vi "read_tiff_header.vi"() -> ()   [LabVIEW 2013]
uses:
  <vilib>/vision/NI_Vision_Development_Module.lvlib
  <vilib>/Analysis/NI_AALPro.lvlib
panel:
  in  "Tab Control":enum32{"Page 1", "Page2", "Page 3", "Page 4"}(tab)
  out "Image":T1(plugin-control)
  out "byte order":T2(ring)
  out "version":u16 format="%x"
  out "byteorder":u16 format="%x"
  in  "frame_index":i32(listbox)
  in  "Directory Entry_index":i32(listbox)
  in  "DE_Data":T3(tab)
  out "type1":u8[](array[numeric])
  out "type2":string
  out "type3":u16[](array[numeric])
  out "type4":u32[](array[numeric])
  out "type5":u32[](array[numeric])
  out "BitDeepth":u32
  out "ImagerWidth":u32
  out "ImageLength":u32
  out "Histogram Graph":T4(graph)
  in  "16-bit Display Mapping:All Elements":T5={"Conversion Method"=2, "Minimum Value"=-30, "Maximum Value"=225, "Number Of Shifts"=0}
  out "tag_ID":u16 format="%x"
  out "DE_data_num":u32
  out "type_ID":u16 format="%x"
  out "DE_data_offset":u32
  out "current_DE_offset":u32 format="%x"
  out "current_IFD_offset":u32 format="%x"
  out "DE_tag_IDs":u16[](array[numeric]) format="%x"
  out "RowsPerStrip":u32
  out "StripByteCounts":u32[](array[numeric])
  out "output array":i32[][](array[numeric])
  out "file header":T6 {"byteorder" format="%x"; "version" format="%x"; "Offset_first_IFD" format="%x"}
  out "DE_num":u16 format="%x"
  out "index of RowsPerStrip":i32
  out "index of bitdeepth":i32
  out "index of StripByteCounts":i32
  out "index of StripOffsets":i32
  out "index of ImageLength":i32
  out "index of ImageWidth":i32
  out "StripOffsets":u32[](array[numeric]) format="%x"
  out "IFD_offset_Array":u32[](array[numeric]) format="%x"
  in  "open":bool
  out "type2_char":string
  out "type1_U8":u8
  out "type4_U32":u32
  out "type5_RATIONAL":u32
  out "type3_U16":u16
  out "selected path":path
  out "tif_file":refnum<file>
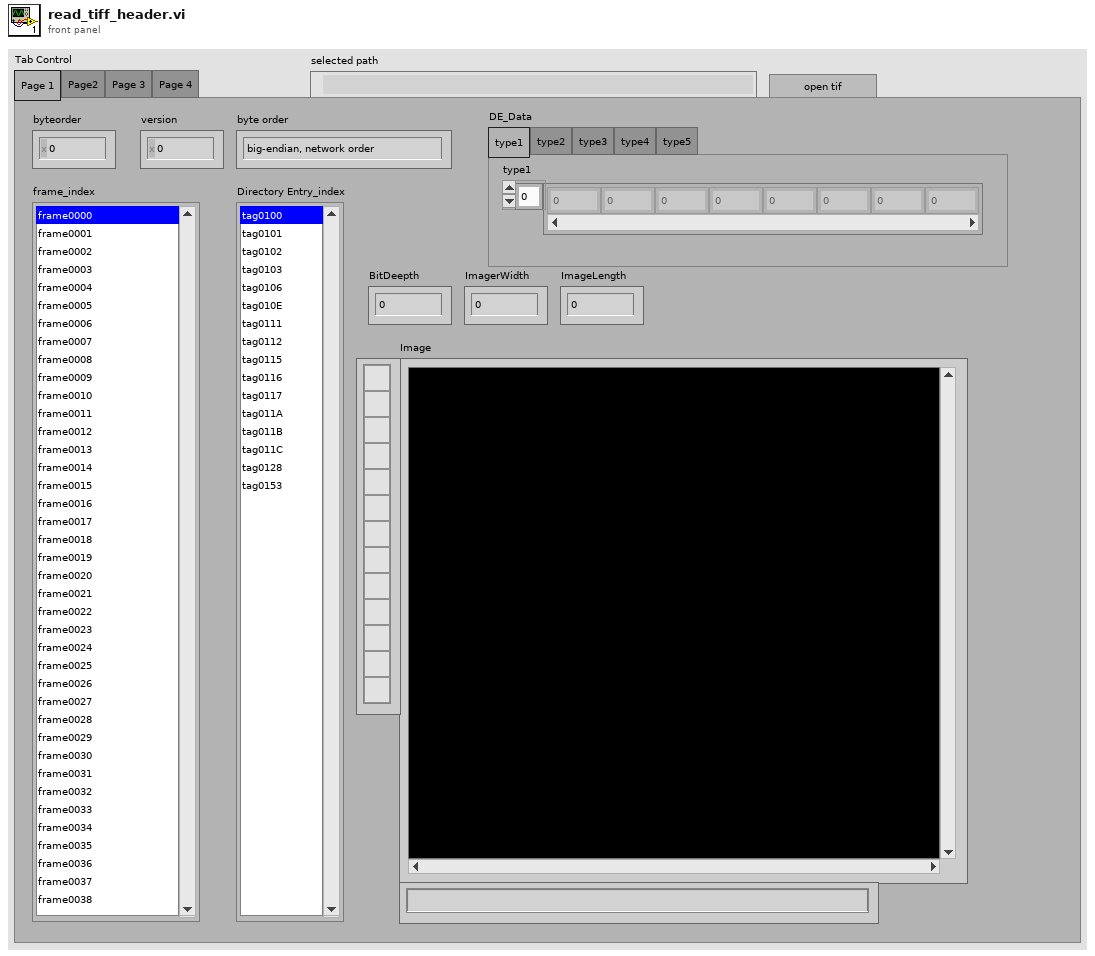
[diagram p1: front panel]
types:
  T1 = typedef "IMAQ Image.ctl" = refnum<image>
  T2 = enum16{"big-endian, network order", "native, host order", "little-endian"}
  T3 = enum32{"type1", "type2", "type3", "type4", "type5"}
  T4 = cluster{"X Values":dbl[], "Histogram: h(x)":i32[]}
  T5 = cluster{"Conversion Method":u32, "Minimum Value":i32, "Maximum Value":i32, "Number Of Shifts":i32}
  T6 = cluster{"byteorder":u16, "version":u16, "Offset_first_IFD":u32}
  T7 = cluster{"tag_ID":u16, "type_ID":u16, "DE_data_num":u32, "DE_data_offset":u32, "type1":u8[], "type2":string, "type3":u16[], "type4":u32[], "type5":u32[]}
  T8 = typedef "Image Type" = u32
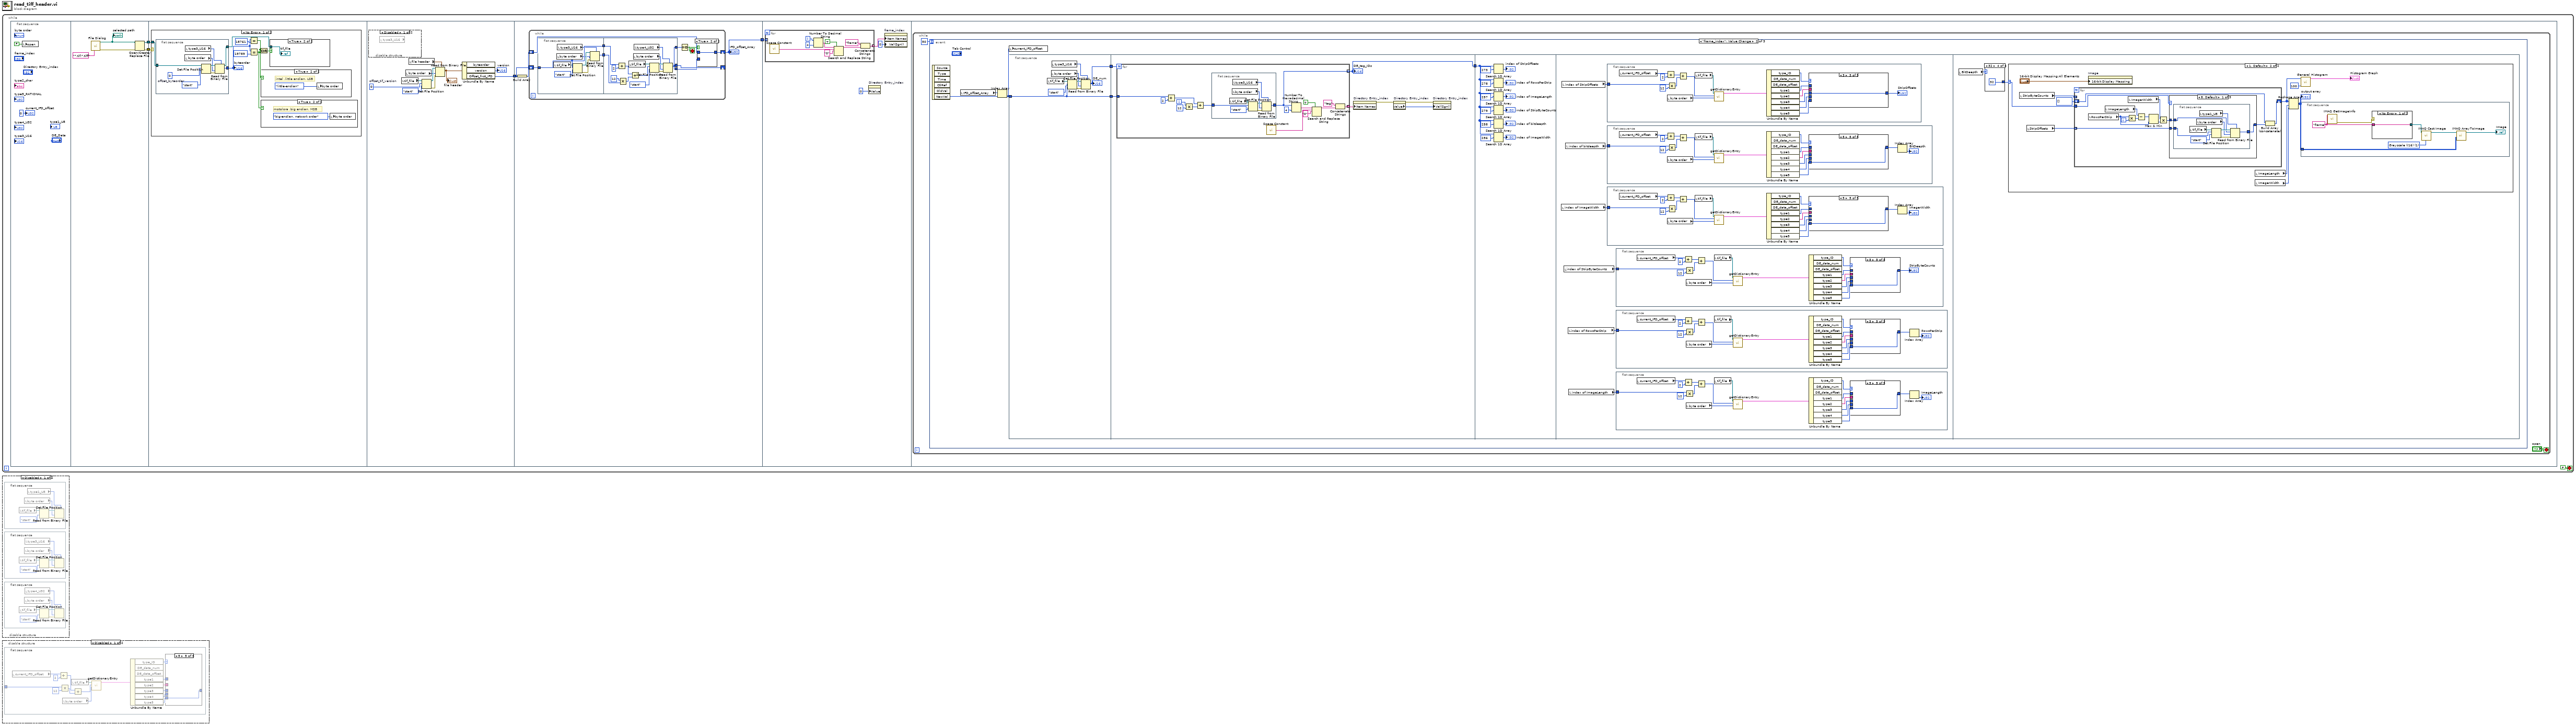
[diagram p0: block diagram]
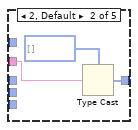
[diagram p3: hidden frame]
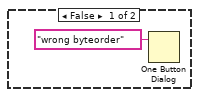
[diagram p7: hidden frame]
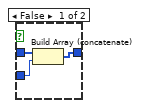
[diagram p12: hidden frame]
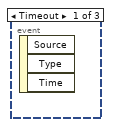
[diagram p13: hidden frame]
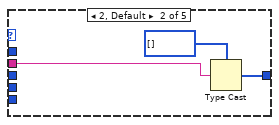
[diagram p15: hidden frame]
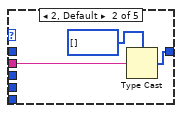
[diagram p19: hidden frame]
diagram:
  n1 = while {
    stop <- FALSE stop-if-true
    n2 = flat-sequence {
      tunnel: [w9] -> w5
      tunnel: [w8] -> w2
      tunnel: w5 -> [w14]
      tunnel: w2 -> [w13]
      tunnel: [w36] -> w1
      tunnel: [w47] -> w4
      tunnel: w1 -> [w46]
      tunnel: w4 -> [w87]
      frame #0 {
        n3 = local write "open"(FALSE ("Stop Button")) -> ()
        "current_IFD_offset" <- u32 0 ("current_IFD_offset")
      }
      frame #1 {
        n4 = call "File Dialog"("pattern (all files)"="*.tif;*.tiff") -> ("selected path"=w10:path, "error out"=w12:errorcluster)  [unwired: 11 in, 2 out]
        "selected path" <- w10
        n5 = Open/Create/Replace File(file path (use dialog)=w10, error in=w12) -> (refnum out=w8:refnum<file>, error out=w9:errorcluster)  [unwired: 4 in, 1 out]
      }
      frame #2 {
        n6 = case shown="No Error" w14 {
          tunnel: w13 -> [w17 _]
          frame No Error {
            n7 = flat-sequence {
              tunnel: [w26] -> w15
              tunnel: w17 -> [w25]
              tunnel: [w24] -> w16
              frame #0 {
                w27 = i64 0  # offset_byteorder
                n8 = local read "byte order"() -> (w28:T2)
                n9 = local read "type3_U16"() -> (w23:u16)
                n10 = Set File Position(offset (in bytes) (0)=w27, refnum=w25, from (0:start)=enum16{"start", "end", "current"}."start") -> (refnum out=w29:refnum<file>, error out=w30:errorcluster)  [unwired: 1 in]
                n11 = Read from Binary File(5:w23, 8:w30, 9:w28, 11:w29) -> (2:w26:u16, 3:w24:refnum<file>)  [unwired: 2 in, 2 out]
              }
            }
            n12 = Equal?(x=w15, y=u16 18761) -> (x = y?=w20:bool)
            n13 = Equal?(x=w15, y=u16 19789) -> (x = y?=w19:bool)
            n14 = Or(x=w20, y=w19) -> (x .or. y?=w18:bool)
            n15 = case shown="True" w20 {
              frame False {
              }
              frame True {
                # "intel ,little endian, LSB"
                n16 = local write "byte order"(T2."little-endian" ("byte order")) -> ()
              }
            }
            n17 = case shown="True" w19 {
              frame False {
              }
              frame True {
                # "motolora ,big endian, MSB"
                n18 = local write "byte order"(T2."big-endian, network order" ("byte order")) -> ()
              }
            }
            n19 = case shown="True" w18 {
              tunnel: w16 -> [_ w33]
              frame False {
                n20 = One Button Dialog(message="wrong byteorder") -> ()  [unwired: 1 in, 1 out]
              }
              frame True {
                "tif_file" <- w33
              }
            }
            "byteorder" <- w15
          }
          frame Error {
          }
        }
      }
      frame #3 {
        w40 = i64 0  # offset_tif_version
        n21 = disable-structure shown="Disabled" {
          frame Disabled {
            n22 = local read "type3_U16"() -> ()  [unwired: 1 out]
          }
          frame Enabled {
          }
        }
        n23 = local read "tif_file"() -> (w45:refnum<file>)
        n24 = local read "byte order"() -> (w41:T2)
        n25 = local read "file header"() -> (w39:T6)
        n26 = Set File Position(offset (in bytes) (0)=w40, refnum=w45, from (0:start)=enum16{"start", "end", "current"}."start") -> (refnum out=w42:refnum<file>, error out=w43:errorcluster)  [unwired: 1 in]
        n27 = Read from Binary File(5:w39, 8:w43, 9:w41, 11:w42) -> (2:w38:T6)  [unwired: 2 in, 3 out]
        "file header" <- w38
        n28 = Unbundle By Name(w38) -> ("version"=→"version":u16, "Offset_first_IFD"=w36:u32)  [unwired: 1 out]
      }
      frame #4 {
        n29 = Build Array(w46) -> (w48:u32[])
        n30 = while {
          shift-right: [w55] -> _
          shift-left: w46 -> [w57]
          shift-right: [w50] -> w47
          shift-left: w48 -> [w51]
          stop <- w49 stop-if-true
          n31 = flat-sequence {
            tunnel: w57 -> [w68]
            tunnel: [w69] -> w54
            tunnel: [w68] -> w53
            tunnel: [w70] -> w56
            tunnel: [w70] -> w55
            tunnel: w54 -> [w72]
            tunnel: w53 -> [w71]
            tunnel: [w70] -> w52
            frame #0 {
              n32 = local read "tif_file"() -> (w67:refnum<file>)
              n33 = local read "byte order"() -> (w63:T2)
              n34 = local read "type3_U16"() -> (w62:u16)
              n35 = Set File Position(offset (in bytes) (0)=w68, refnum=w67, from (0:start)=enum16{"start", "end", "current"}."start") -> (refnum out=w64:refnum<file>, error out=w65:errorcluster)  [unwired: 1 in]
              n36 = Read from Binary File(5:w62, 8:w65, 9:w63, 11:w64) -> (2:w69:u16)  [unwired: 2 in, 3 out]
            }
            frame #1 {
              n37 = Add(x=w71, y=u32 2) -> (x+y=w75:u32)
              n38 = Multiply(x=u16 12 ("y"), y=w72) -> (x*y=w74:u16)
              n39 = local read "tif_file"() -> (w83:refnum<file>)
              n40 = Add(x=w75, y=w74) -> (x+y=w73:u32)
              n41 = local read "byte order"() -> (w79:T2)
              n42 = local read "type4_U32"() -> (w78:u32)
              n43 = Set File Position(offset (in bytes) (0)=w73, refnum=w83, from (0:start)=enum16{"start", "end", "current"}."start") -> (refnum out=w80:refnum<file>, error out=w81:errorcluster)  [unwired: 1 in]
              n44 = Read from Binary File(5:w78, 8:w81, 9:w79, 11:w80) -> (2:w70:u32)  [unwired: 2 in, 3 out]
            }
          }
          n45 = Equal To 0?(x=w56) -> (x = 0?=w49:bool)
          n46 = case shown="True" w49 {
            tunnel: w52 -> [w60 _]
            tunnel: w51 -> [w59 w61]
            tunnel: [w58 w61] -> w50
            frame False {
              n47 = Build Array (concatenate)(w59, w60) -> (w58:u32[])
            }
            frame True {
            }
          }
        }
        "IFD_offset_Array" <- w47
      }
      frame #5 {
        n48 = for {
          tunnel: w87 -> [_] mode=indexing
          tunnel: [w90] -> w86 mode=indexing
          i -> [w96]
          n49 = call <vilib>:"Space Constant.vi"() -> ("String"=w92:string)
          n50 = Number To Decimal String(number=w96, width (-)=i16 4) -> (decimal integer string=w93:string)
          n51 = Search and Replace String(replace all?=TRUE ("replace all? (F)"), input string=w93, search string=w92, replace string="0" ("replace string (\"\")")) -> (result string=w88:string)  [unwired: 4 in, 3 out]
          n52 = Concatenate Strings("frame" ("string"), w88) -> (w90:string)
        }
        n53 = property on="Directory Entry_index" class="LstBox (strict)"("Value"=0 ("Value (Signaling)")) -> ()  [unwired: 2 in, 2 out]
        n54 = property on="frame_index" class="LstBox (strict)"("Item Names"=w86, "Val(Sgnl)"=0 ("Value (Signaling)")) -> ()  [unwired: 2 in, 2 out]
      }
      frame #6 {
        n55 = while {
          stop <- "open" stop-if-true
          n56 = event shown="[1] \"frame_index\": Value Change" {
            selector: _ -> [_ _ _]
            dyn-events: _ -> [_ _ _]
            timeout: 50 -> [_ _ _]
            event Timeout {
              n57 = event-data() -> ()  [unwired: 1 in, 3 out]
            }
            event "frame_index": Value Change {
              n58 = event-data() -> ("NewVal"=w103:i32)  [unwired: 1 in, 5 out]
              n59 = local read "IFD_offset_Array"() -> (w104:u32[])
              n60 = Index Array(array=w104, index=w103) -> (element=w102:u32)
              n61 = local write "current_IFD_offset"(w102) -> ()
              n62 = flat-sequence {
                tunnel: w102 -> [w105]
                tunnel: [w106] -> w101
                tunnel: [w105] -> w100
                tunnel: w101 -> [w119]
                tunnel: w100 -> [w114]
                tunnel: [w113] -> w99
                tunnel: w99 -> [w144]
                frame #0 {
                  n63 = local read "tif_file"() -> (w112:refnum<file>)
                  n64 = local read "byte order"() -> (w108:T2)
                  n65 = local read "type3_U16"() -> (w107:u16)
                  n66 = Set File Position(offset (in bytes) (0)=w105, refnum=w112, from (0:start)=enum16{"start", "end", "current"}."start") -> (refnum out=w109:refnum<file>, error out=w110:errorcluster)  [unwired: 1 in]
                  n67 = Read from Binary File(5:w107, 8:w110, 9:w108, 11:w109) -> (2:w106:u16)  [unwired: 2 in, 3 out]
                  "DE_num" <- w106
                }
                frame #1 {
                  n68 = for {
                    N: w119 -> [_]
                    tunnel: [w128] -> w118 mode=indexing
                    tunnel: w114 -> [w127]
                    tunnel: [w120] -> w113 mode=indexing
                    i -> [w125]
                    n69 = Add(x=w127, y=u32 2) -> (x+y=w123:u32)
                    n70 = Multiply(x=w125, y=12) -> (x*y=w122:i32)
                    n71 = Add(x=w123, y=w122) -> (x+y=w121:u32)
                    n72 = flat-sequence {
                      tunnel: w121 -> [w137]
                      tunnel: [w136] -> w120
                      frame #0 {
                        n73 = local read "tif_file"() -> (w143:refnum<file>)
                        n74 = local read "byte order"() -> (w139:T2)
                        n75 = local read "type3_U16"() -> (w138:u16)
                        n76 = Set File Position(offset (in bytes) (0)=w137, refnum=w143, from (0:start)=enum16{"start", "end", "current"}."start") -> (refnum out=w140:refnum<file>, error out=w141:errorcluster)  [unwired: 1 in]
                        n77 = Read from Binary File(5:w138, 8:w141, 9:w139, 11:w140) -> (2:w136:u16)  [unwired: 2 in, 3 out]
                      }
                    }
                    n78 = call <vilib>:"Space Constant.vi"() -> ("String"=w132:string)
                    n79 = Number To Hexadecimal String(1:i16 4 ("width (-)"), 2:w120) -> (0:w133:string)
                    n80 = Search and Replace String(replace all?=TRUE ("replace all? (F)"), input string=w133, search string=w132, replace string="0" ("replace string (\"\")")) -> (result string=w129:string)  [unwired: 4 in, 3 out]
                    n81 = Concatenate Strings("tag" ("string"), w129) -> (w128:string)
                  }
                  "DE_tag_IDs" <- w113
                  n82 = property on="Directory Entry_index" class="LstBox (strict)"("Item Names"=w118) -> (error out=w116:errorcluster)  [unwired: 2 in, 1 out]
                  n83 = property on="Directory Entry_index" class="LstBox (strict)"(error in=w116) -> (error out=w115:errorcluster, "Value"=w117:i32)  [unwired: 1 in, 1 out]
                  n84 = property on="Directory Entry_index" class="LstBox (strict)"(error in=w115, "Val(Sgnl)"=w117) -> ()  [unwired: 1 in, 2 out]
                }
                frame #2 {
                  n85 = Search 1D Array(1D array=w144, element=u16 273) -> (index of element=→"index of StripOffsets":i32)  [unwired: 1 in]
                  n86 = Search 1D Array(1D array=w144, element=u16 278) -> (index of element=→"index of RowsPerStrip":i32)  [unwired: 1 in]
                  n87 = Search 1D Array(1D array=w144, element=u16 257) -> (index of element=→"index of ImageLength":i32)  [unwired: 1 in]
                  n88 = Search 1D Array(1D array=w144, element=u16 279) -> (index of element=→"index of StripByteCounts":i32)  [unwired: 1 in]
                  n89 = Search 1D Array(1D array=w144, element=u16 258) -> (index of element=→"index of bitdeepth":i32)  [unwired: 1 in]
                  n90 = Search 1D Array(1D array=w144, element=u16 256) -> (index of element=→"index of ImageWidth":i32)  [unwired: 1 in]
                }
                frame #3 {
                  n91 = local read "index of ImageWidth"() -> (w159:i32)
                  n92 = local read "index of StripOffsets"() -> (w157:i32)
                  n93 = local read "index of StripByteCounts"() -> (w160:i32)
                  n94 = local read "index of bitdeepth"() -> (w162:i32)
                  n95 = local read "index of RowsPerStrip"() -> (w161:i32)
                  n96 = local read "index of ImageLength"() -> (w158:i32)
                  n97 = flat-sequence {
                    tunnel: w157 -> [w177]
                    frame #0 {
                      n98 = local read "current_IFD_offset"() -> (w179:u32)
                      n99 = Add(x=w179, y=2) -> (x+y=w175:u32)
                      n100 = local read "byte order"() -> (w171:T2)
                      n101 = Multiply(x=w177, y=12) -> (x*y=w174:i32)
                      n102 = Add(x=w175, y=w174) -> (x+y=w173:u32)
                      n103 = local read "tif_file"() -> (w172:refnum<file>)
                      n104 = call "getDictionaryEntry.vi"("byte order"=w171, "DE_offset"=w173, "tif_file"=w172) -> ("output cluster"=w170:T7)  [unwired: 7 in, 1 out]
                      n105 = Unbundle By Name(w170) -> ("type_ID"=w169:u16, "type1"=w168:u8[], "type2"=w164:string, "type3"=w167:u16[], "type4"=w166:u32[], "type5"=w165:u32[])  [unwired: 2 out]
                      n106 = case shown="3" w169 {
                        tunnel: [w180 w181 w184 w185 w186] -> w163
                        tunnel: w168 -> [w180 _ _ _ _]
                        tunnel: w167 -> [_ _ w184 _ _]
                        tunnel: w166 -> [_ _ _ w185 _]
                        tunnel: w165 -> [_ _ _ _ w186]
                        tunnel: w164 -> [_ w183 _ _ _]
                        frame 1 {
                        }
                        frame 2, Default {
                          n107 = Type Cast(type=u8[] [] ("type1"), x=w183) -> (*(type *) &x=w181:u8[])
                        }
                        frame 3 {
                        }
                        frame 4 {
                        }
                        frame 5 {
                        }
                      }
                      "StripOffsets" <- w163
                    }
                  }
                  n108 = flat-sequence {
                    tunnel: w162 -> [w301]
                    frame #0 {
                      n109 = local read "current_IFD_offset"() -> (w303:u32)
                      n110 = Add(x=w303, y=2) -> (x+y=w299:u32)
                      n111 = local read "byte order"() -> (w295:T2)
                      n112 = Multiply(x=w301, y=12) -> (x*y=w298:i32)
                      n113 = Add(x=w299, y=w298) -> (x+y=w297:u32)
                      n114 = local read "tif_file"() -> (w296:refnum<file>)
                      n115 = call "getDictionaryEntry.vi"("byte order"=w295, "DE_offset"=w297, "tif_file"=w296) -> ("output cluster"=w294:T7)  [unwired: 7 in, 1 out]
                      n116 = Unbundle By Name(w294) -> ("type_ID"=w293:u16, "type1"=w292:u8[], "type2"=w288:string, "type3"=w291:u16[], "type4"=w290:u32[], "type5"=w289:u32[])  [unwired: 2 out]
                      n117 = case shown="5" w293 {
                        tunnel: [w304 w305 w308 w309 w310] -> w287
                        tunnel: w292 -> [w304 _ _ _ _]
                        tunnel: w291 -> [_ _ w308 _ _]
                        tunnel: w290 -> [_ _ _ w309 _]
                        tunnel: w289 -> [_ _ _ _ w310]
                        tunnel: w288 -> [_ w307 _ _ _]
                        frame 1 {
                        }
                        frame 2, Default {
                          n118 = Type Cast(type=u8[] [] ("type1"), x=w307) -> (*(type *) &x=w305:u8[])
                        }
                        frame 3 {
                        }
                        frame 4 {
                        }
                        frame 5 {
                        }
                      }
                      n119 = Index Array(array=w287) -> (element=→"BitDeepth":u32)  [unwired: 1 in]
                    }
                  }
                  n120 = flat-sequence {
                    tunnel: w159 -> [w227]
                    frame #0 {
                      n121 = local read "current_IFD_offset"() -> (w229:u32)
                      n122 = Add(x=w229, y=2) -> (x+y=w225:u32)
                      n123 = local read "byte order"() -> (w221:T2)
                      n124 = Multiply(x=w227, y=12) -> (x*y=w224:i32)
                      n125 = Add(x=w225, y=w224) -> (x+y=w223:u32)
                      n126 = local read "tif_file"() -> (w222:refnum<file>)
                      n127 = call "getDictionaryEntry.vi"("byte order"=w221, "DE_offset"=w223, "tif_file"=w222) -> ("output cluster"=w220:T7)  [unwired: 7 in, 1 out]
                      n128 = Unbundle By Name(w220) -> ("type_ID"=w219:u16, "type1"=w218:u8[], "type2"=w214:string, "type3"=w217:u16[], "type4"=w216:u32[], "type5"=w215:u32[])  [unwired: 2 out]
                      n129 = case shown="5" w219 {
                        tunnel: [w230 w231 w234 w235 w236] -> w213
                        tunnel: w218 -> [w230 _ _ _ _]
                        tunnel: w217 -> [_ _ w234 _ _]
                        tunnel: w216 -> [_ _ _ w235 _]
                        tunnel: w215 -> [_ _ _ _ w236]
                        tunnel: w214 -> [_ w233 _ _ _]
                        frame 1 {
                        }
                        frame 2, Default {
                          n130 = Type Cast(type=u8[] [] ("type1"), x=w233) -> (*(type *) &x=w231:u8[])
                        }
                        frame 3 {
                        }
                        frame 4 {
                        }
                        frame 5 {
                        }
                      }
                      n131 = Index Array(array=w213) -> (element=→"ImagerWidth":u32)  [unwired: 1 in]
                    }
                  }
                  n132 = flat-sequence {
                    tunnel: w160 -> [w251]
                    frame #0 {
                      n133 = local read "current_IFD_offset"() -> (w253:u32)
                      n134 = Add(x=w253, y=2) -> (x+y=w249:u32)
                      n135 = Multiply(x=w251, y=12) -> (x*y=w248:i32)
                      n136 = local read "byte order"() -> (w245:T2)
                      n137 = Add(x=w249, y=w248) -> (x+y=w247:u32)
                      n138 = local read "tif_file"() -> (w246:refnum<file>)
                      n139 = call "getDictionaryEntry.vi"("byte order"=w245, "DE_offset"=w247, "tif_file"=w246) -> ("output cluster"=w244:T7)  [unwired: 7 in, 1 out]
                      n140 = Unbundle By Name(w244) -> ("type_ID"=w243:u16, "type1"=w242:u8[], "type2"=w238:string, "type3"=w241:u16[], "type4"=w240:u32[], "type5"=w239:u32[])  [unwired: 2 out]
                      n141 = case shown="5" w243 {
                        tunnel: [w254 w255 w258 w259 w260] -> w237
                        tunnel: w242 -> [w254 _ _ _ _]
                        tunnel: w241 -> [_ _ w258 _ _]
                        tunnel: w240 -> [_ _ _ w259 _]
                        tunnel: w239 -> [_ _ _ _ w260]
                        tunnel: w238 -> [_ w257 _ _ _]
                        frame 1 {
                        }
                        frame 2, Default {
                          n142 = Type Cast(type=u8[] [] ("type1"), x=w257) -> (*(type *) &x=w255:u8[])
                        }
                        frame 3 {
                        }
                        frame 4 {
                        }
                        frame 5 {
                        }
                      }
                      "StripByteCounts" <- w237
                    }
                  }
                  n143 = flat-sequence {
                    tunnel: w161 -> [w276]
                    frame #0 {
                      n144 = local read "current_IFD_offset"() -> (w278:u32)
                      n145 = Add(x=w278, y=2) -> (x+y=w274:u32)
                      n146 = Multiply(x=w276, y=12) -> (x*y=w273:i32)
                      n147 = local read "byte order"() -> (w270:T2)
                      n148 = Add(x=w274, y=w273) -> (x+y=w272:u32)
                      n149 = local read "tif_file"() -> (w271:refnum<file>)
                      n150 = call "getDictionaryEntry.vi"("byte order"=w270, "DE_offset"=w272, "tif_file"=w271) -> ("output cluster"=w269:T7)  [unwired: 7 in, 1 out]
                      n151 = Unbundle By Name(w269) -> ("type_ID"=w268:u16, "type1"=w267:u8[], "type2"=w263:string, "type3"=w266:u16[], "type4"=w265:u32[], "type5"=w264:u32[])  [unwired: 2 out]
                      n152 = case shown="5" w268 {
                        tunnel: [w279 w280 w283 w284 w285] -> w262
                        tunnel: w267 -> [w279 _ _ _ _]
                        tunnel: w266 -> [_ _ w283 _ _]
                        tunnel: w265 -> [_ _ _ w284 _]
                        tunnel: w264 -> [_ _ _ _ w285]
                        tunnel: w263 -> [_ w282 _ _ _]
                        frame 1 {
                        }
                        frame 2, Default {
                          n153 = Type Cast(type=u8[] [] ("type1"), x=w282) -> (*(type *) &x=w280:u8[])
                        }
                        frame 3 {
                        }
                        frame 4 {
                        }
                        frame 5 {
                        }
                      }
                      n154 = Index Array(array=w262) -> (element=→"RowsPerStrip":u32)  [unwired: 1 in]
                    }
                  }
                  n155 = flat-sequence {
                    tunnel: w158 -> [w202]
                    frame #0 {
                      n156 = local read "current_IFD_offset"() -> (w204:u32)
                      n157 = Add(x=w204, y=2) -> (x+y=w200:u32)
                      n158 = Multiply(x=w202, y=12) -> (x*y=w199:i32)
                      n159 = local read "byte order"() -> (w196:T2)
                      n160 = Add(x=w200, y=w199) -> (x+y=w198:u32)
                      n161 = local read "tif_file"() -> (w197:refnum<file>)
                      n162 = call "getDictionaryEntry.vi"("byte order"=w196, "DE_offset"=w198, "tif_file"=w197) -> ("output cluster"=w195:T7)  [unwired: 7 in, 1 out]
                      n163 = Unbundle By Name(w195) -> ("type_ID"=w194:u16, "type1"=w193:u8[], "type2"=w189:string, "type3"=w192:u16[], "type4"=w191:u32[], "type5"=w190:u32[])  [unwired: 2 out]
                      n164 = case shown="5" w194 {
                        tunnel: [w205 w206 w209 w210 w211] -> w188
                        tunnel: w193 -> [w205 _ _ _ _]
                        tunnel: w192 -> [_ _ w209 _ _]
                        tunnel: w191 -> [_ _ _ w210 _]
                        tunnel: w190 -> [_ _ _ _ w211]
                        tunnel: w189 -> [_ w208 _ _ _]
                        frame 1 {
                        }
                        frame 2, Default {
                          n165 = Type Cast(type=u8[] [] ("type1"), x=w208) -> (*(type *) &x=w206:u8[])
                        }
                        frame 3 {
                        }
                        frame 4 {
                        }
                        frame 5 {
                        }
                      }
                      n166 = Index Array(array=w188) -> (element=→"ImageLength":u32)  [unwired: 1 in]
                    }
                  }
                }
                frame #4 {
                  n167 = local read "BitDeepth"() -> (w312:u32)
                  n168 = case shown="32" w312 {
                    tunnel: [0 8 16 32] -> w311
                    frame 0, Default {
                    }
                    frame 8 {
                    }
                    frame 16 {
                    }
                    frame 32 {
                    }
                  }
                  n169 = case shown="1, Default" w311 {
                    selector: w311 -> [_ w321]
                    frame 0 {
                    }
                    frame 1, Default {
                      n170 = local read "StripByteCounts"() -> (w323:u32[])
                      n171 = local read "StripOffsets"() -> (w322:u32[])
                      n172 = for {
                        tunnel: w323 -> [_] mode=indexing
                        tunnel: w322 -> [w339] mode=indexing
                        tunnel: w321 -> [w335]
                        shift-right: [w336] -> w316
                        shift-left: i32[] [] -> [w337]
                        i -> [w345]
                        n173 = local read "RowsPerStrip"() -> (w342:u32)
                        n174 = local read "ImageLength"() -> (w343:u32)
                        n175 = Multiply(x=w342, y=w345) -> (x*y=w344:u32)
                        n176 = local read "ImagerWidth"() -> (w346:u32)
                        n177 = Subtract(x=w343, y=w344) -> (x-y=w340:u32)
                        n178 = Max & Min(x=w340, y=w342) -> (min(x,y)=w341:u32)  [unwired: 1 out]
                        n179 = Multiply(x=w346, y=w341) -> (x*y=w334:u32)
                        n180 = case shown="8, Default" w335 {
                          tunnel: w339 -> [w349 w361 w373]
                          tunnel: [w347 w359 w372] -> w338
                          tunnel: w334 -> [w348 w360 w371]
                          frame 8, Default {
                            n181 = flat-sequence {
                              tunnel: w349 -> [w352]
                              tunnel: w348 -> [w351]
                              tunnel: [w350] -> w347
                              frame #0 {
                                n182 = local read "tif_file"() -> (w358:refnum<file>)
                                n183 = local read "byte order"() -> (w354:T2)
                                n184 = local read "type1_U8"() -> (w353:u8)
                                n185 = Set File Position(offset (in bytes) (0)=w352, refnum=w358, from (0:start)=enum16{"start", "end", "current"}."start") -> (refnum out=w355:refnum<file>, error out=w356:errorcluster)  [unwired: 1 in]
                                n186 = Read from Binary File(5:w353, 8:w356, 9:w354, 10:w351, 11:w355) -> (2:w350:u8[])  [unwired: 1 in, 3 out]
                              }
                            }
                          }
                          frame 16 {
                            n187 = flat-sequence {
                              tunnel: w361 -> [w365]
                              tunnel: w360 -> [w364]
                              tunnel: [w363] -> w359
                              frame #0 {
                                n188 = local read "tif_file"() -> (w370:refnum<file>)
                                n189 = local read "byte order"() -> (w366:T2)
                                n190 = Set File Position(offset (in bytes) (0)=w365, refnum=w370, from (0:start)=enum16{"start", "end", "current"}."start") -> (refnum out=w367:refnum<file>, error out=w368:errorcluster)  [unwired: 1 in]
                                n191 = Read from Binary File(5:i16 0, 8:w368, 9:w366, 10:w364, 11:w367) -> (2:w363:i16[])  [unwired: 1 in, 3 out]
                              }
                            }
                          }
                          frame 32 {
                            n192 = flat-sequence {
                              tunnel: w373 -> [w377]
                              tunnel: w371 -> [w376]
                              tunnel: [w375] -> w372
                              frame #0 {
                                n193 = local read "tif_file"() -> (w382:refnum<file>)
                                n194 = local read "byte order"() -> (w378:T2)
                                n195 = Set File Position(offset (in bytes) (0)=w377, refnum=w382, from (0:start)=enum16{"start", "end", "current"}."start") -> (refnum out=w379:refnum<file>, error out=w380:errorcluster)  [unwired: 1 in]
                                n196 = Read from Binary File(5:0, 8:w380, 9:w378, 10:w376, 11:w379) -> (2:w375:i32[])  [unwired: 1 in, 3 out]
                              }
                            }
                          }
                        }
                        n197 = Build Array (concatenate)(w337, w338) -> (w336:i32[])
                      }
                      n198 = property on="Image" class="ImageControl"("16-bit Display Mapping"="16-bit Display Mapping:All Elements") -> ()  [unwired: 2 in, 2 out]
                      n199 = local read "ImageLength"() -> (w317:u32)
                      n200 = local read "ImagerWidth"() -> (w318:u32)
                      n201 = Reshape Array(w316, w317, w318) -> (w319:i32[][])
                      "output array" <- w319
                      n202 = call <vilib>:"General Histogram.vi"("X"=w316, "# bins"=100) -> ("Histogram Graph"=→"Histogram Graph":T4)  [unwired: 9 in, 4 out]
                      n203 = flat-sequence {
                        tunnel: w319 -> [w324]
                        frame #0 {
                          w328 = T8 1 items=["Grayscale (U8)", "Grayscale (I16)", "Grayscale (SGL)", "Complex (CSG)", "RGB (U32)", "HSL (U32)", "RGB (U64)", "Grayscale (U16)"] ("Image Type")
                          w330 = "frame" ("Image Name")
                          n204 = call "IMAQ GetImageInfo"("Image"=w330) -> ("error out"=w329:errorcluster)  [unwired: 3 in, 7 out]
                          n205 = case shown="No Error" w329 {
                            tunnel: w330 -> [w331 w333]
                            tunnel: [w331 w332] -> w327
                            frame No Error {
                            }
                            frame Error {
                              n206 = call "IMAQ Create"("Image Name"=w333) -> ("New Image"=w332:T1)  [unwired: 4 in, 1 out]
                            }
                          }
                          n207 = call "IMAQ Cast Image"("Image Type"=w328, "Image Src"=w327) -> ("Image Dst Out"=w326:T1)  [unwired: 8 in, 1 out]
                          n208 = call "IMAQ ArrayToImage"("Image Pixels (I16)"=w324, "Image"=w326) -> ("Image Out"=→"Image":T1)  [unwired: 8 in, 1 out]
                        }
                      }
                    }
                  }
                }
              }
            }
            event "Directory Entry_index": Value Change {
              n209 = event-data() -> ("NewVal"=w399:i32)  [unwired: 1 in, 5 out]
              n210 = flat-sequence {
                tunnel: w399 -> [w407]
                tunnel: [w403] -> w398
                tunnel: [w401] -> w397
                frame #0 {
                  n211 = local read "current_IFD_offset"() -> (w409:u32)
                  n212 = Add(x=w409, y=2) -> (x+y=w405:u32)
                  n213 = Multiply(x=w407, y=12) -> (x*y=w404:i32)
                  n214 = local read "byte order"() -> (w400:T2)
                  n215 = local read "tif_file"() -> (w402:refnum<file>)
                  n216 = Add(x=w405, y=w404) -> (x+y=w403:u32)
                  n217 = call "getDictionaryEntry.vi"("byte order"=w400, "DE_offset"=w403, "tif_file"=w402) -> ("output cluster"=w401:T7)  [unwired: 7 in, 1 out]
                }
              }
              n218 = Unbundle By Name(w397) -> ("tag_ID"=→"tag_ID":u16, "type_ID"=w394:u16, "DE_data_num"=→"DE_data_num":u32, "DE_data_offset"=→"DE_data_offset":u32, "type1"=→"type1":u8[], "type2"=→"type2":string, "type3"=→"type3":u16[], "type4"=→"type4":u32[], "type5"=→"type5":u32[])
              "type_ID" <- w394
              n219 = Decrement(x=w394) -> (x-1=w396:u16)
              n220 = property on="DE_Data" class="TabCtl (strict)"("Value"=w396) -> ()  [unwired: 2 in, 2 out]
              "current_DE_offset" <- w398
            }
          }
        }
      }
    }
  }
  n221 = disable-structure shown="Disabled" {
    frame Disabled {
      n222 = flat-sequence {
        frame #0 {
          n223 = local read "tif_file"() -> (w427:refnum<file>)
          n224 = local read "byte order"() -> (w423:T2)
          n225 = local read "type1_U8"() -> (w422:u8)
          n226 = Set File Position(refnum=w427, from (0:start)=enum16{"start", "end", "current"}."start") -> (refnum out=w424:refnum<file>, error out=w425:errorcluster)  [unwired: 2 in]
          n227 = Read from Binary File(5:w422, 8:w425, 9:w423, 11:w424) -> ()  [unwired: 2 in, 4 out]
        }
      }
      n228 = flat-sequence {
        frame #0 {
          n229 = local read "tif_file"() -> (w421:refnum<file>)
          n230 = local read "byte order"() -> (w417:T2)
          n231 = local read "type3_U16"() -> (w416:u16)
          n232 = Set File Position(refnum=w421, from (0:start)=enum16{"start", "end", "current"}."start") -> (refnum out=w418:refnum<file>, error out=w419:errorcluster)  [unwired: 2 in]
          n233 = Read from Binary File(5:w416, 8:w419, 9:w417, 11:w418) -> ()  [unwired: 2 in, 4 out]
        }
      }
      n234 = flat-sequence {
        frame #0 {
          n235 = local read "tif_file"() -> (w415:refnum<file>)
          n236 = local read "byte order"() -> (w411:T2)
          n237 = local read "type4_U32"() -> (w410:u32)
          n238 = Set File Position(refnum=w415, from (0:start)=enum16{"start", "end", "current"}."start") -> (refnum out=w412:refnum<file>, error out=w413:errorcluster)  [unwired: 2 in]
          n239 = Read from Binary File(5:w410, 8:w413, 9:w411, 11:w412) -> ()  [unwired: 2 in, 4 out]
        }
      }
    }
    frame Enabled {
    }
  }
  n240 = disable-structure shown="Disabled" {
    frame Disabled {
      n241 = flat-sequence {
        tunnel: _ -> [w441]
        frame #0 {
          n242 = local read "current_IFD_offset"() -> (w443:u32)
          n243 = Add(x=w443, y=2) -> (x+y=w439:u32)
          n244 = Multiply(x=w441, y=12) -> (x*y=w438:i32)
          n245 = local read "byte order"() -> (w435:T2)
          n246 = local read "tif_file"() -> (w436:refnum<file>)
          n247 = Add(x=w439, y=w438) -> (x+y=w437:u32)
          n248 = call "getDictionaryEntry.vi"("byte order"=w435, "DE_offset"=w437, "tif_file"=w436) -> ("output cluster"=w434:T7)  [unwired: 7 in, 1 out]
          n249 = Unbundle By Name(w434) -> ("type_ID"=w433:u16, "type1"=w432:u8[], "type2"=w428:string, "type3"=w431:u16[], "type4"=w430:u32[], "type5"=w429:u32[])  [unwired: 2 out]
          n250 = case shown="5" w433 {
            tunnel: [w444 w445 w448 w449 w450] -> _
            tunnel: w432 -> [w444 _ _ _ _]
            tunnel: w431 -> [_ _ w448 _ _]
            tunnel: w430 -> [_ _ _ w449 _]
            tunnel: w429 -> [_ _ _ _ w450]
            tunnel: w428 -> [_ w447 _ _ _]
            frame 1 {
            }
            frame 2, Default {
              n251 = Type Cast(type=u8[] [] ("type1"), x=w447) -> (*(type *) &x=w445:u8[])
            }
            frame 3 {
            }
            frame 4 {
            }
            frame 5 {
            }
          }
        }
      }
    }
    frame Enabled {
    }
  }
